vi "ziSync.vi"(0 "Handle In":T1 {"Handle" format="0x%08x"; "Conn" format="0x%08x"}, 11 "Error In":errorcluster) -> (4 "Handle Out":T1 {"Handle" format="0x%08x"; "Conn" format="0x%08x"}, 15 "Error Out":errorcluster)   [LabVIEW 2018, in "Zurich Instruments LabOne.lvlib"]
doc: "Syncs all the settings on the device and flushes all buffers."
uses:
  Zurich Instruments LabOne.lvlib
  ziTypeHandle.ctl
  ziLV32.dll
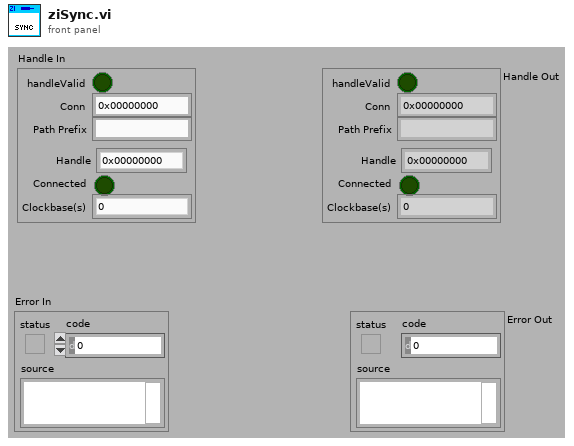
[diagram p1: front panel]
types:
  T1 = typedef "Zurich Instruments LabOne.lvlib/ziTypeHandle.ctl" = cluster{"handleValid":bool, "Conn":u64, "Path Prefix":string, "Handle":u64, "Connected":bool, "Clockbase(s)":dbl}
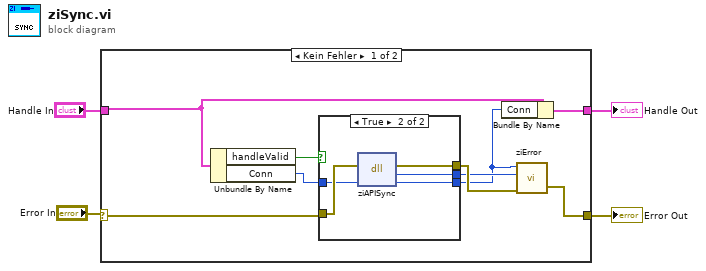
[diagram p0: block diagram]
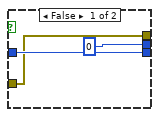
[diagram p2: hidden frame]
diagram:
  n1 = case shown="Kein Fehler" "Error In" {
    selector: "Error In" -> [w7 w23]
    tunnel: [w12 w23] -> w4
    tunnel: [w8 w22] -> w3
    tunnel: "Handle In" -> [w6 w22]
    frame No Error {
      n2 = Unbundle By Name(w6) -> ("handleValid"=w9:bool, "Conn"=w13:u64)
      n3 = case shown="True" w9 {
        tunnel: w7 -> [w15 w21]
        tunnel: w13 -> [w16 w20]
        tunnel: [w15 w19] -> w11
        tunnel: [u32 0 ("return type") w18] -> w10
        tunnel: [w16 w17] -> w5
        frame False {
        }
        frame True {
          n4 = dll-call lib="ziLV*.*" fn="ziAPISync"(error in=w21, "Conn"=w20) -> (error out=w19:errorcluster, "return type"=w18:u32, "Conn"=w17:u64)  [unwired: 2 in, 1 out]
        }
      }
      n5 = Bundle By Name(cluster=w6, "Conn"=w5) -> (w8:T1)
      n6 = call "ziError.vi"("Conn"=w5, "ziErrorCode"=w10, "Error In"=w11) -> ("Error Out"=w12:errorcluster)  [unwired: 2 in, 1 out]
    }
    frame Error {
    }
  }
  "Error Out" <- w4
  "Handle Out" <- w3
